vi "GPIB ConvBox Protocol FG.vi"(7 "Action":T1, 8 "error in (no error)":errorcluster, 10 "GPIB ConvBox Config":T2={"Port"="Com1", "ConvBox Address"="", "Assert Ren with IFC"=FALSE, "System controller"=TRUE, "IST bit sense"=TRUE, "GPIB Address"="1"}, 11 "Device Item Ref in":T3 format="%.0x") -> (0 "error out":errorcluster, 2 "GPIB ConvBox Config":T2={"Port"="Com1", "ConvBox Address"="", "Assert Ren with IFC"=FALSE, "System controller"=TRUE, "IST bit sense"=TRUE, "GPIB Address"="1"}, 3 "Item Ref out":T3 format="%.0x")   [LabVIEW 2019, in "Instrument Addon Shared.lvlib"]
uses:
  Instrument Addon Shared.lvlib
  <vilib>/NI VeriStand/Custom Device API/Custom Device Item Ref.ctl
  Types/GPIB ConvBox Settings.ctl
  Types/FG Control.ctl
  Constants.vi
  <vilib>/NI VeriStand/Custom Device API/Get Item Property (Boolean).vi
  <vilib>/NI VeriStand/Custom Device API/Get Item Property (String).vi
  <vilib>/NI VeriStand/Custom Device API/Set Item Property (Boolean).vi
  <vilib>/NI VeriStand/Custom Device API/Set Item Property (String).vi
  <vilib>/NI VeriStand/Custom Device API/Custom Device API.lvlib
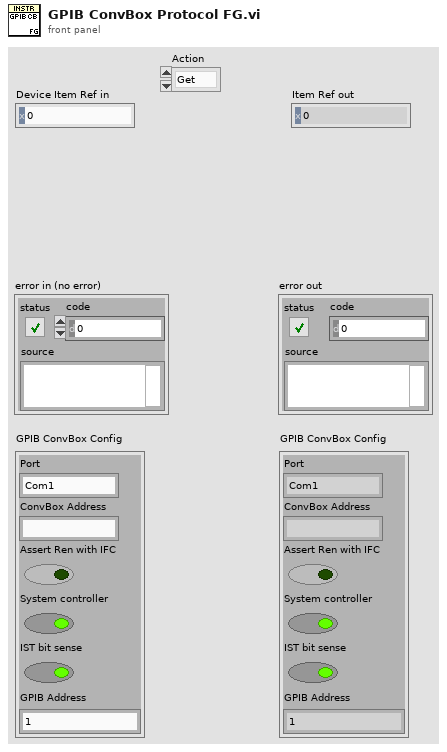
[diagram p1: front panel]
types:
  T1 = typedef "Instrument Addon Shared.lvlib/FG Control.ctl" = enum16{"Get", "Set"}
  T2 = typedef "Instrument Addon Shared.lvlib/GPIB ConvBox Settings.ctl" = cluster{"Port":string, "ConvBox Address":string, "Assert Ren with IFC":bool, "System controller":bool, "IST bit sense":bool, "GPIB Address":string}
  T3 = typedef "Custom Device API.lvlib/Custom Device Item Ref.ctl" = u64
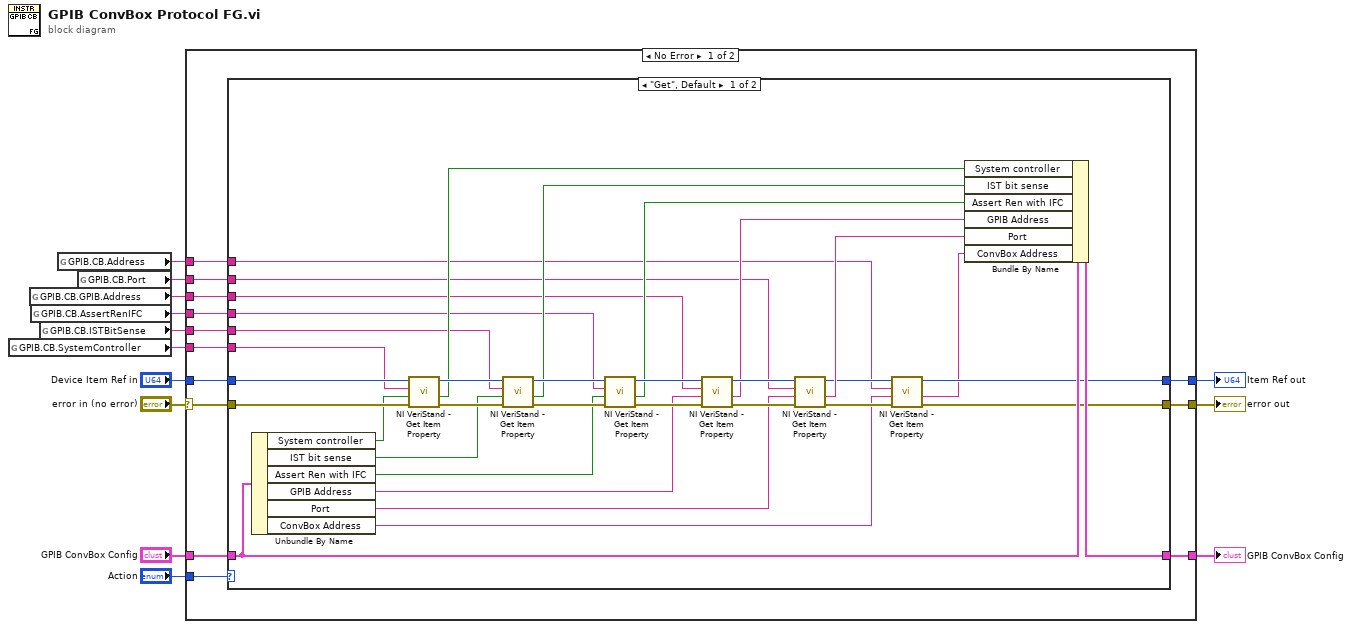
[diagram p0: block diagram]
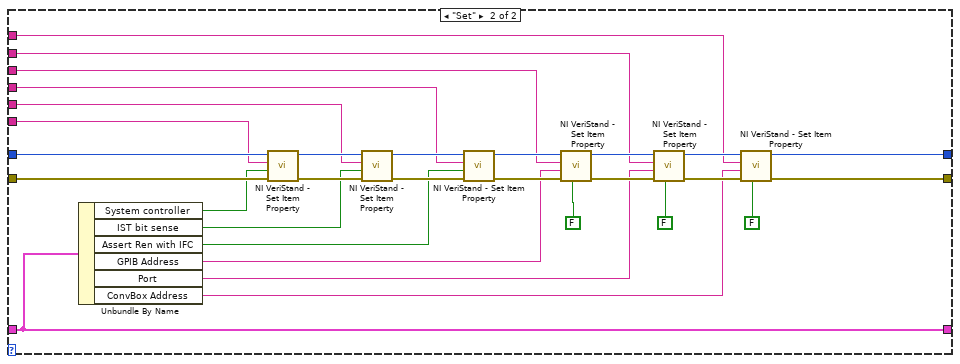
[diagram p2: hidden frame]
diagram:
  n1 = global read "Constants.vi" "GPIB.CB.SystemController"() -> (w2:string)
  n2 = global read "Constants.vi" "GPIB.CB.GPIB.Address"() -> (w5:string)
  n3 = global read "Constants.vi" "GPIB.CB.AssertRenIFC"() -> (w4:string)
  n4 = global read "Constants.vi" "GPIB.CB.ISTBitSense"() -> (w3:string)
  n5 = global read "Constants.vi" "GPIB.CB.Address"() -> (w1:string)
  n6 = global read "Constants.vi" "GPIB.CB.Port"() -> (w13:string)
  n7 = case shown="No Error" "error in (no error)" {
    selector: "error in (no error)" -> [w21 w93]
    tunnel: w13 -> [w26 _]
    tunnel: [w25 w91] -> w12
    tunnel: "Device Item Ref in" -> [w24 w91]
    tunnel: "GPIB ConvBox Config" -> [w23 w92]
    tunnel: [w22 w93] -> w9
    tunnel: [w20 w92] -> w7
    tunnel: "Action" -> [w19 _]
    tunnel: w5 -> [w18 _]
    tunnel: w4 -> [w17 _]
    tunnel: w3 -> [w16 _]
    tunnel: w2 -> [w15 _]
    tunnel: w1 -> [w14 _]
    frame No Error {
      n8 = case shown="\"Get\", Default" w19 {
        tunnel: w26 -> [w40 w70]
        tunnel: [w31 w64] -> w25
        tunnel: w24 -> [w59 w81]
        tunnel: w23 -> [w39 w80]
        tunnel: [w32 w63] -> w22
        tunnel: w21 -> [w60 w82]
        tunnel: [w49 w80] -> w20
        tunnel: w18 -> [w41 w74]
        tunnel: w17 -> [w42 w73]
        tunnel: w16 -> [w43 w72]
        tunnel: w15 -> [w44 w71]
        tunnel: w14 -> [w28 w61]
        frame "Get", Default {
          n9 = Unbundle By Name(w39) -> ("System controller"=w38:bool, "IST bit sense"=w37:bool, "Assert Ren with IFC"=w36:bool, "GPIB Address"=w35:string, "Port"=w34:string, "ConvBox Address"=w29:string)
          n10 = call-poly <vilib>:"NI VeriStand - Get Item Property.vi"("error in (no error)"=w60, "Default Value"=w38, "Property Name"=w44, "Item Ref in"=w59) -> ("error out"=w58:errorcluster, "Value"=w45:bool, "Item Ref out"=w54:T3)  [unwired: 4 in, 1 out]
          n11 = call-poly <vilib>:"NI VeriStand - Get Item Property.vi"("error in (no error)"=w58, "Default Value"=w37, "Property Name"=w43, "Item Ref in"=w54) -> ("error out"=w57:errorcluster, "Value"=w46:bool, "Item Ref out"=w53:T3)  [unwired: 4 in, 1 out]
          n12 = call-poly <vilib>:"NI VeriStand - Get Item Property.vi"("error in (no error)"=w57, "Default Value"=w36, "Property Name"=w42, "Item Ref in"=w53) -> ("error out"=w56:errorcluster, "Value"=w47:bool, "Item Ref out"=w52:T3)  [unwired: 4 in, 1 out]
          n13 = call-poly <vilib>:"NI VeriStand - Get Item Property.vi"("error in (no error)"=w56, "Default Value"=w35, "Property Name"=w41, "Item Ref in"=w52) -> ("error out"=w55:errorcluster, "Value"=w48:string, "Item Ref out"=w51:T3)  [unwired: 4 in, 1 out]
          n14 = call-poly <vilib>:"NI VeriStand - Get Item Property.vi"("error in (no error)"=w55, "Default Value"=w34, "Property Name"=w40, "Item Ref in"=w51) -> ("error out"=w33:errorcluster, "Value"=w50:string, "Item Ref out"=w30:T3)  [unwired: 4 in, 1 out]
          n15 = call-poly <vilib>:"NI VeriStand - Get Item Property.vi"("error in (no error)"=w33, "Default Value"=w29, "Property Name"=w28, "Item Ref in"=w30) -> ("error out"=w32:errorcluster, "Value"=w27:string, "Item Ref out"=w31:T3)  [unwired: 4 in, 1 out]
          n16 = Bundle By Name(cluster=w39, "System controller"=w45, "IST bit sense"=w46, "Assert Ren with IFC"=w47, "GPIB Address"=w48, "Port"=w50, "ConvBox Address"=w27) -> (w49:T2)
        }
        frame "Set" {
          n17 = Unbundle By Name(w80) -> ("System controller"=w75:bool, "IST bit sense"=w76:bool, "Assert Ren with IFC"=w77:bool, "GPIB Address"=w78:string, "Port"=w79:string, "ConvBox Address"=w62:string)
          n18 = call-poly <vilib>:"NI VeriStand - Set Item Property.vi"("error in (no error)"=w82, "Value"=w75, "Property Name"=w71, "Item Ref in"=w81) -> ("error out"=w90:errorcluster, "Item Ref out"=w86:T3)  [unwired: 5 in, 1 out]
          n19 = call-poly <vilib>:"NI VeriStand - Set Item Property.vi"("error in (no error)"=w90, "Value"=w76, "Property Name"=w72, "Item Ref in"=w86) -> ("error out"=w89:errorcluster, "Item Ref out"=w85:T3)  [unwired: 5 in, 1 out]
          n20 = call-poly <vilib>:"NI VeriStand - Set Item Property.vi"("error in (no error)"=w89, "Value"=w77, "Property Name"=w73, "Item Ref in"=w85) -> ("error out"=w88:errorcluster, "Item Ref out"=w84:T3)  [unwired: 5 in, 1 out]
          n21 = call-poly <vilib>:"NI VeriStand - Set Item Property.vi"("Binary String (T)"=FALSE, "error in (no error)"=w88, "Value"=w78, "Property Name"=w74, "Item Ref in"=w84) -> ("error out"=w87:errorcluster, "Item Ref out"=w83:T3)  [unwired: 4 in, 1 out]
          n22 = call-poly <vilib>:"NI VeriStand - Set Item Property.vi"("Binary String (T)"=FALSE, "error in (no error)"=w87, "Value"=w79, "Property Name"=w70, "Item Ref in"=w83) -> ("error out"=w66:errorcluster, "Item Ref out"=w65:T3)  [unwired: 4 in, 1 out]
          n23 = call-poly <vilib>:"NI VeriStand - Set Item Property.vi"("Binary String (T)"=FALSE, "error in (no error)"=w66, "Value"=w62, "Property Name"=w61, "Item Ref in"=w65) -> ("error out"=w63:errorcluster, "Item Ref out"=w64:T3)  [unwired: 4 in, 1 out]
        }
      }
    }
    frame Error {
    }
  }
  "Item Ref out" <- w12
  "error out" <- w9
  "GPIB ConvBox Config" <- w7
